vi "PKG_IMC_SetPassword.vi"(0 "handle":u32, 1 "pwnlen":i8, 2 "rpwlen":string, 5 "oldpassword":string, 7 "pwolen":i8, 9 "password":string, 12 "rPW":string) -> (3 "function return":i32, 4 "handle out":u32, 6 "oldpassword out":string, 8 "rpwlen out":string, 10 "password out":string, 14 "rPW out":string)   [LabVIEW 2011, in "IMC_Pkg4xxx.lvlib"]
doc: "PKG_IMC_SetPassword(IMC_HANDLE handle, char* oldpassword, char pwolen, char* password, char pwnlen, char rPW[128], char *rpwlen);"
uses:
  IMC_Pkg4xxx.lvlib
  IMC_Pkg4xxx.dll
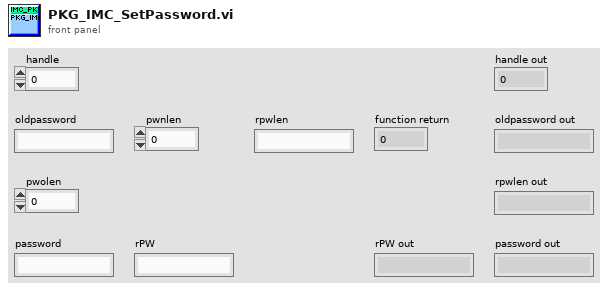
[diagram p1: front panel]
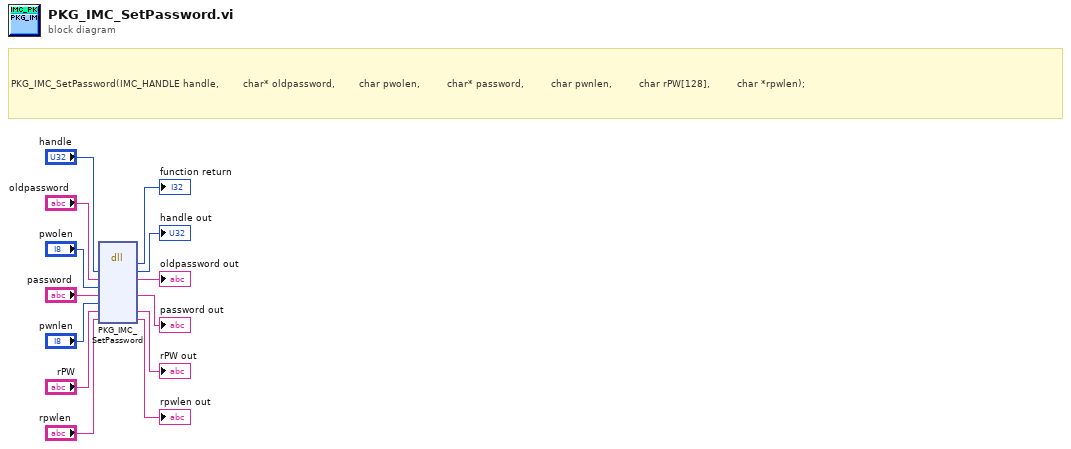
[diagram p0: block diagram]
diagram:
  # "PKG_IMC_SetPassword(IMC_HANDLE handle,  \t\t\t\t\t\tchar* oldpassword,\t\t\t\t\t\t\t\tchar pwolen,\t\t\t\t\t\t\t\t\tchar* password,\t\t\t\t\t\t\t\t\tchar pwnlen,\t\t\t\t\t\t\t\t\tchar rPW[128],\t\t\t\t\t\t\t\t\tchar *rpwlen);"
  n1 = dll-call lib="PTH1mabs F光盘刻录\niMC MotionIMCNet_V4.0IMCAppincLabviewIMC_PKG4xxxIMC_PKG4xxx\nIMC_Pkg4xxx.*" fn="PKG_IMC_SetPassword"("handle"="handle", "oldpassword"="oldpassword", "pwolen"="pwolen", "password"="password", "pwnlen"="pwnlen", "rPW"="rPW", "rpwlen"="rpwlen") -> (→"function return":i32, "handle"=→"handle out":u32, "oldpassword"=→"oldpassword out":string, "password"=→"password out":string, "rPW"=→"rPW out":string, "rpwlen"=→"rpwlen out":string)  [unwired: 5 in, 2 out]
